vi "update.vi"(8 "error in (no error)":errorcluster, 10 "data":dbl, 11 "node in":refnum<class "node.lvclass">) -> (0 "error out":errorcluster, 3 "node out":refnum<class "node.lvclass">)   [LabVIEW 2014, in "Linked List.lvlib" / "node.lvclass"]
uses:
  node.lvclass
  node.lvclass/node.ctl
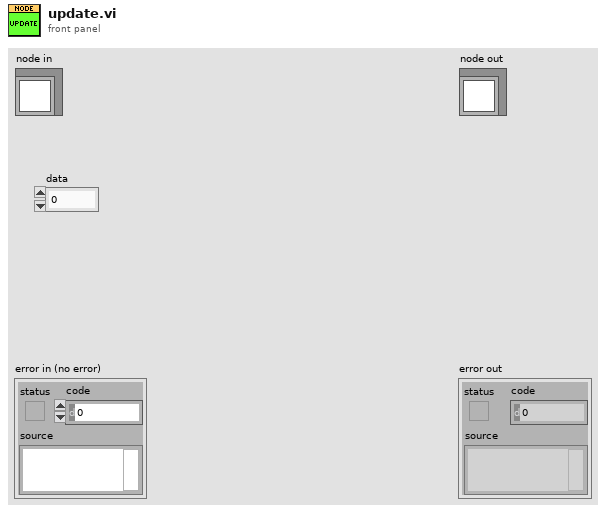
[diagram p1: front panel]
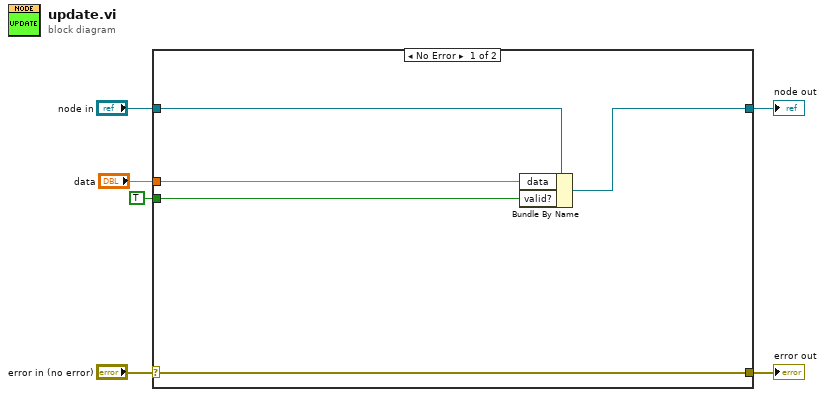
[diagram p0: block diagram]
diagram:
  n1 = case shown="No Error" "error in (no error)" {
    selector: "error in (no error)" -> [w11 w13]
    tunnel: [w11 w13] -> w5
    tunnel: [w9 w12] -> w3
    tunnel: "node in" -> [w10 w12]
    tunnel: "data" -> [w8 _]
    tunnel: TRUE ("valid?") -> [w7 _]
    frame No Error {
      n2 = Bundle By Name(cluster=w10, "data"=w8, "valid?"=w7) -> (w9:refnum<class "node.lvclass">)
    }
    frame Error {
    }
  }
  "error out" <- w5
  "node out" <- w3
